vi "Sensors.vi"(11 "Error In":errorcluster) -> (3 "Error Out":errorcluster)   [LabVIEW 2019]
uses:
  <vilib>/Platform/TimedLoop/XDataNode/timing_clust.ctl
  <vilib>/Platform/TimedLoop/XDataNode/nitl_modes.ctl
  <vilib>/Platform/TimedLoop/XDataNode/wakeup.ctl
  Global.vi
  <vilib>/Utility/error.llb/Error Cluster From Error Code.vi
  <vilib>/myRIO/Common/Instrument Driver Framework/myRIO v1.0/AI/vis/myRIO v1.0 Read AI.vi
  <vilib>/Platform/TimedLoop/XDataNode/XDataNode.xnode
  <vilib>/myRIO/Instrument Drivers/Onboard IO/AI/AI.lvlib
  <vilib>/Platform/TimedLoop/XDataNode/XDNodeRunTimeDep.lvlib
panel:
  in  "Period [s]":dbl=0.001
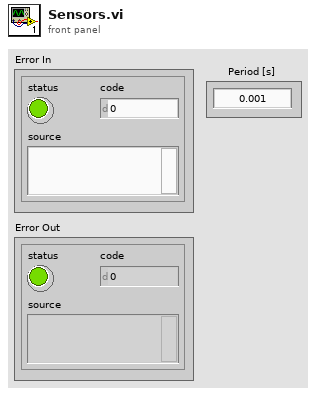
[diagram p1: front panel]
types:
  T1 = typedef "XDNodeRunTimeDep.lvlib/timing_clust.ctl" = cluster{"Expected End [f-1]":u64, "Actual End [f-1]":u64, "Finished Late? [f-1]":bool, "Expected End [i-1]":u64, "Actual End [i-1]":u64, "Finished Late? [i-1]":bool, "Expected Start [i]":u64, "Actual Start [i]":u64, "Expected Start [f]":u64, "Actual Start [f]":u64, "Source Name":string, "Structure Name":string, "Period":i64, "Deadline":i64, "Offset":i64, "Start":i64, "Priority":i32, "Timeout":i32, "Mode":T2, "Wakeup Reason":T3, "Error":errorcluster, "Source Type":string, "Secondary Source Type":string, "Global End Time":u64, "Global Start Time":u64, "Frame Duration":u64, "Iteration Duration":u64, "Assigned CPU":i32, "I/O Scan Engine Mode":u32}
  T2 = typedef "XDNodeRunTimeDep.lvlib/nitl_modes.ctl" = enum32{"No Change", "Process missed periods, maintain original phase", "Discard missed periods, maintain original phase", "Process missed periods, ignore original phase", "Discard missed periods, ignore original phase"}
  T3 = typedef "XDNodeRunTimeDep.lvlib/wakeup.ctl" = enum32{"Normal", "Aborted", "Asynchronous wakeup", "Timing source error", "Timed loop error", "Timeout"}
  T4 = typedef "AI.lvlib/AI Reference.ctl" = cluster{"myRIO Reference":T5, "AI Channels List":T9, "AI Scaling Constants List":T11}
  T5 = typedef "myRIO Generic Hardware Reference.ctl" = cluster{"myRIO Model":T6, "myRIO Hardware Reference":T7}
  T6 = typedef "Hardware Version Enum.ctl" = enum16{"Unknown", "myRIO-1900", "myRIO-1950", "roboRIO", "NI ELVIS RIO CM", "ELVIS III"}
  T7 = typedef "myRIO v1.0 Reference.ctl" = cluster{"Generic FPGA Reference":T8, "Allow multiple opens":bool}
  T8 = typedef "Generic FPGA Reference.ctl" = refnum<k20>
  T9 = typedef "AI Channels List.ctl" = T10[]
  T10 = typedef "AI Channels Enum.ctl" = enum16{"Not Connected", "AudioIn/Left", "AudioIn/Right", "C/AI0", "C/AI1", "A/AI0", "A/AI1", "A/AI2", "A/AI3", "A/AI4", "A/AI5", "A/AI6", "A/AI7", "B/AI0", "B/AI1", "B/AI2", "B/AI3", "B/AI4", "B/AI5", "B/AI6", "B/AI7", "AI/AI0", "AI/AI1", "AI/AI2", "AI/AI3", "A/AI0 (DIFF)", "A/AI1 (DIFF)", "A/AI2 (DIFF)", "A/AI3 (DIFF)", "B/AI0 (DIFF)", "B/AI1 (DIFF)", "B/AI2 (DIFF)", "B/AI3 (DIFF)"}
  T11 = typedef "Analog Scaling Constants List.ctl" = T12[]
  T12 = typedef "Analog Scaling Constants.ctl" = cluster{"LSB Weight (Volts)":dbl, "Offset (Volts)":dbl, "Signed?":bool}
  T13 = cluster{"dbl Scaled Value":dbl, "dbl Scaled Value":dbl}
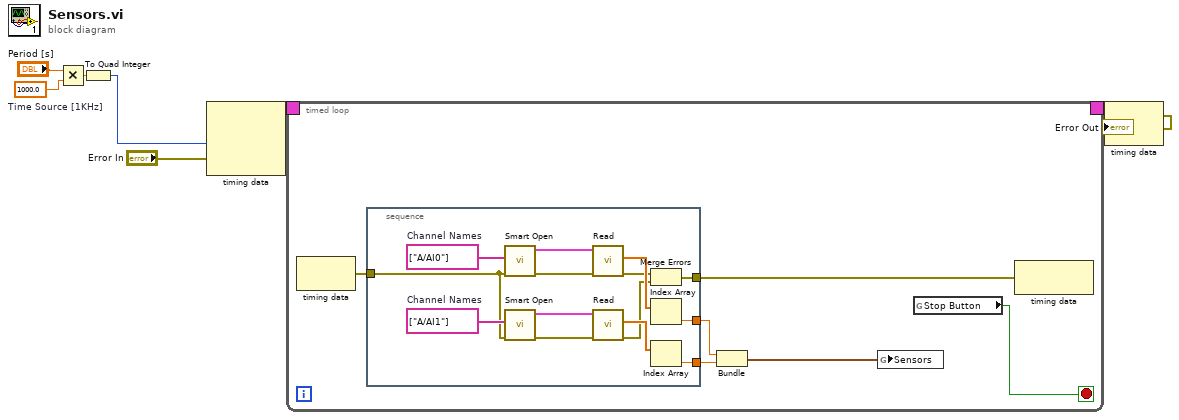
[diagram p0: block diagram]
diagram:
  w3 = 1000.0  # Time Source [1KHz]
  n1 = Multiply(x="Period [s]", y=w3) -> (x*y=w2:dbl)
  n2 = To Quad Integer(1:w2) -> (0:w1:i64)
  n3 = node-c288(w1, "Error In") -> (w8:T1)  [unwired: 1 in]
  n4 = timed-loop {
    timing: w8 -> [_]
    timing-out: [_] -> w7
    stop <- w11 stop-if-true
    n5 = node-c288() -> (w13:errorcluster)  [unwired: 1 in]
    n6 = stacked-sequence {
      tunnel: w13 -> [w19]
      tunnel: [w26] -> w10
      tunnel: [w16] -> w12
      tunnel: [w15] -> w14
      frame #0 {
        w20 = tag[] ["A/AI1"]  # Channel Names
        w24 = tag[] ["A/AI0"]  # Channel Names
        n7 = call <vilib>:"Smart Open.vi"("error in (no error)"=w19, "Channel Names"=w24) -> ("error out"=w28:errorcluster, "AI Ref Out"=w27:T4)  [unwired: 8 in]
        n8 = call <vilib>:"Smart Open.vi"("error in (no error)"=w19, "Channel Names"=w20) -> ("error out"=w23:errorcluster, "AI Ref Out"=w22:T4)  [unwired: 8 in]
        n9 = call <vilib>:"Read.vi"("error in (no error)"=w28, "AI Ref In"=w27) -> ("error out"=w17:errorcluster, "Values"=w25:dbl[])  [unwired: 7 in, 1 out]
        n10 = call <vilib>:"Read.vi"("error in (no error)"=w23, "AI Ref In"=w22) -> ("error out"=w18:errorcluster, "Values"=w21:dbl[])  [unwired: 7 in, 1 out]
        n11 = Merge Errors(w17, w18) -> (w16:errorcluster)
        n12 = Index Array(array=w25) -> (element=w26:dbl)  [unwired: 1 in]
        n13 = Index Array(array=w21) -> (element=w15:dbl)  [unwired: 1 in]
      }
    }
    n14 = Bundle("dbl Scaled Value"=w10, "dbl Scaled Value"=w14) -> (w9:T13)  [unwired: 1 in]
    n15 = global write "Global.vi" "Sensors"(w9) -> ()
    n16 = global read "Global.vi" "Stop Button"() -> (w11:bool)
    n17 = node-c288(w12) -> ()  [unwired: 1 out]
  }
  n18 = node-c288(w7) -> (→"Error Out":errorcluster)
